vi "icListen 2 Response.vi"() -> ()   [LabVIEW 2020, in "PAM Library.lvlib"]
uses:
  PAM Library.lvlib
panel:
  in  "icListen 2 Response":string="Initialization Complete"
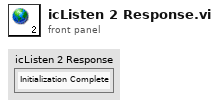
[diagram p1: front panel]
diagram:
